vi "Clear PlotConfig.vi"(8 "error in (no error)":errorcluster, 11 "BluePlotHandle in":refnum<class "RocketPlotHandle.lvclass">) -> (0 "error out":errorcluster, 3 "BluePlotHandle out":refnum<class "RocketPlotHandle.lvclass">)   [LabVIEW 2021, in "RocketPlotHandle.lvclass"]
doc: "Load plot configuration into the attached plot instance.\n\nNote that this will load ALL plot settings from the input \"plot config\" cluster input.\nThere is no mechanism for specifying only a subset of these settings to be loaded.\nIt's all or nothin'\n\nIf you ever needed to modify/load only 1 aspect of a plot, then I recommend:\n- perform \"get plot config\"\n- perform in-place modification of the plot config cluster to adjust what you want to specifically change\n- perform \"load plot config\""
uses:
  RocketPlotHandle.lvclass
  RocketPlotHandle.lvclass/RocketPlotHandle.ctl
  TypeDefs/plot handle queue data.ctl
  TypeDefs/Plot QSM action.ctl
  RocketPlot.lvlib
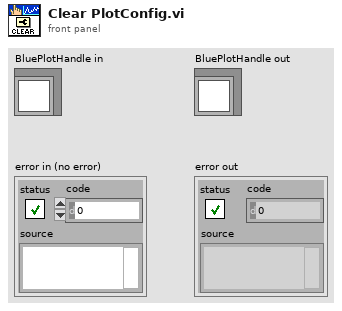
[diagram p1: front panel]
types:
  T1 = typedef "RocketPlot.lvlib/Plot QSM action.ctl" = enum16{"Get Config", "Load Config", "Set TimeToPlot", "Clear Config"}
  T2 = typedef "RocketPlot.lvlib/plot handle queue data.ctl" = cluster{"action":T1, "data":variant}
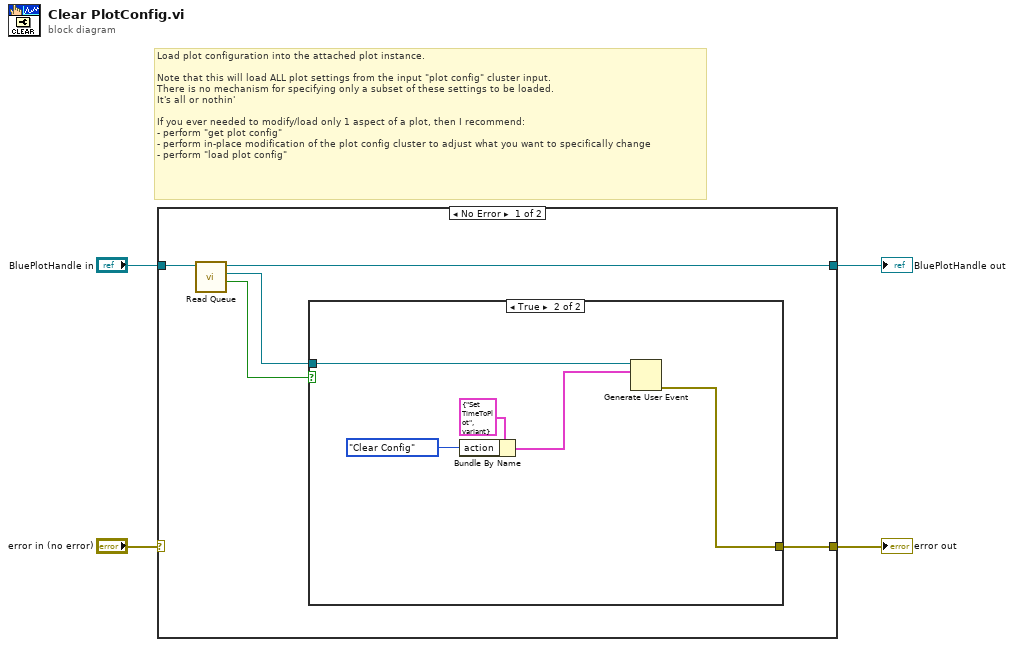
[diagram p0: block diagram]
diagram:
  # "Load plot configuration into the attached plot instance.\n\nNote that this will load ALL plot settings from the input \"plot config\" cluster input.\nThere is no mechanism for specifying only a subset of these settings to be loaded.\nIt's all or nothin'\n\nIf you ever needed to modify/load only 1 aspect of a plot, then I recommend:\n- perform \"get plot config\"\n- perform in-place modification of the plot config cluster to adjust what you want to specifically change\n- perform \"load plot config\""
  n1 = case shown="No Error" "error in (no error)" {
    selector: "error in (no error)" -> [_ w16]
    tunnel: "BluePlotHandle in" -> [w8 w15]
    tunnel: [w5 w16] -> w3
    tunnel: [w6 w15] -> w1
    frame No Error {
      n2 = call "Read Queue.vi"("BluePlotHandle in"=w8) -> ("Valid?"=w9:bool, "UE"=w7:refnum<user-event>, "BluePlotHandle out"=w6:refnum<class "RocketPlotHandle.lvclass">)  [unwired: 8 in]
      n3 = case shown="True" w9 {
        tunnel: w7 -> [_ w14]
        tunnel: [_ w10] -> w5
        frame False {
        }
        frame True {
          n4 = Bundle By Name(cluster=T2 {"action"=enum."Set TimeToPlot", "data"=variant} ("element"), "action"=Plot_QSM_action."Clear Config") -> (w11:T2)
          n5 = Generate User Event(user event=w14, event data cluster=w11) -> (error out=w10:errorcluster)  [unwired: 2 in, 1 out]
        }
      }
    }
    frame Error {
    }
  }
  "BluePlotHandle out" <- w1
  "error out" <- w3
